vi "Kr.vi"(0 "u[k]":dbl, 1 "K":dbl, 2 "tau":dbl, 3 "error in (no error)":errorcluster, 4 "dt":dbl) -> (5 "y[k+1]":dbl, 6 "error out":errorcluster)   [LabVIEW 2019]
uses:
  discrete_control_memory.vi
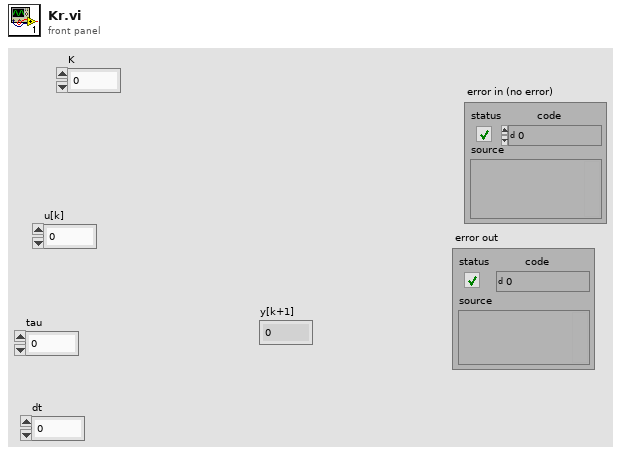
[diagram p1: front panel]
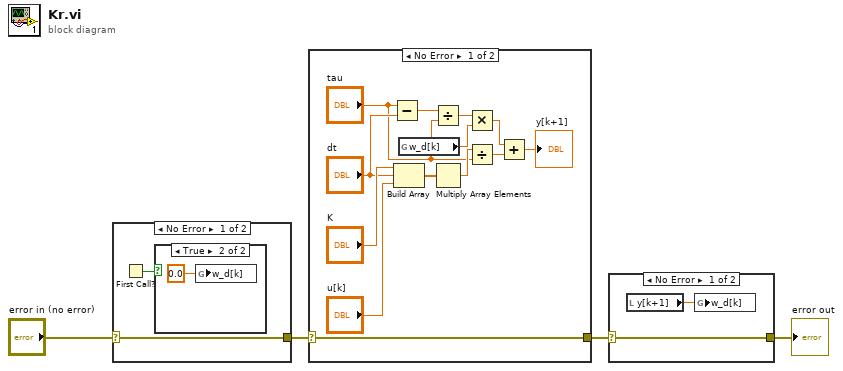
[diagram p0: block diagram]
diagram:
  n1 = case shown="No Error" "error in (no error)" {
    selector: "error in (no error)" -> [w5 w8]
    tunnel: [w5 w8] -> w3
    frame No Error {
      n2 = First Call?() -> (First Call?: T/F=w6:bool)
      n3 = case shown="True" w6 {
        frame False {
        }
        frame True {
          n4 = global write "discrete_control_memory.vi" "w_d[k]"(0.0 ("w_d[k]")) -> ()
        }
      }
    }
    frame Error {
    }
  }
  n5 = case shown="No Error" w3 {
    selector: w3 -> [w21 w22]
    tunnel: [w21 w22] -> w2
    frame No Error {
      n6 = Subtract(x="tau", y="dt") -> (x-y=w20:dbl)
      n7 = Build Array("K", "dt", "u[k]") -> (w12:dbl[])
      n8 = global read "discrete_control_memory.vi" "w_d[k]"() -> (w18:dbl)
      n9 = Divide(x=w20, y="tau") -> (x/y=w19:dbl)
      n10 = Multiply Array Elements(1:w12) -> (0:w11:dbl)
      n11 = Multiply(x=w19, y=w18) -> (x*y=w17:dbl)
      n12 = Divide(x=w11, y="tau") -> (x/y=w9:dbl)
      n13 = Add(x=w17, y=w9) -> (x+y=→"y[k+1]":dbl)
    }
    frame Error {
    }
  }
  n14 = case shown="No Error" w2 {
    selector: w2 -> [w23 w25]
    tunnel: [w23 w25] -> w1
    frame No Error {
      n15 = local read "y[k+1]"() -> (w24:dbl)
      n16 = global write "discrete_control_memory.vi" "w_d[k]"(w24) -> ()
    }
    frame Error {
    }
  }
  "error out" <- w1
